vi "Rotation.vi"(1 "Uncorrected Speed":dbl=-0.0, 2 "Moving Laterally":bool) -> (0 "Output Speed":dbl=-0.0)   [LabVIEW 2013]
uses:
  Robot Global Data.vi
panel:
  in  "Output Range":cluster{"output high":dbl, "output low":dbl}={"output high"=0.4, "output low"=-0.4}
  in  "Gain":dbl=0.02
  in  "Rate Limit (deg/s)":dbl=15.0
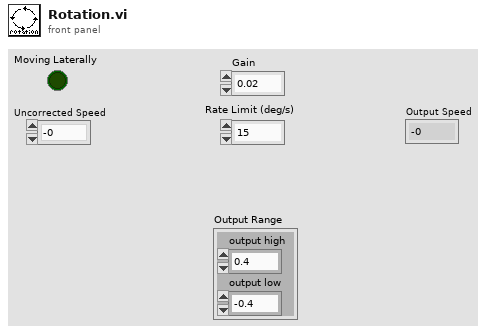
[diagram p1: front panel]
types:
  T1 = typedef "WPI_GyroDevRef.ctl" = cluster{"DevStatus":errorcluster, "Analog Module":T2, "Analog Channel":T3, "Offset":dbl, "Gain (VoltsPerDegree/Second)":dbl}
  T2 = typedef "FPGA_TypedefAnalogModule.ctl" = enum16{"Analog Module 1", "Analog Module 2"}
  T3 = typedef "FPGA_AIChannel.ctl" = enum8{"AI 1", "AI 2", "AI 3", "AI 4", "AI 5", "AI 6", "AI 7", "AI 8", "Invalid"}
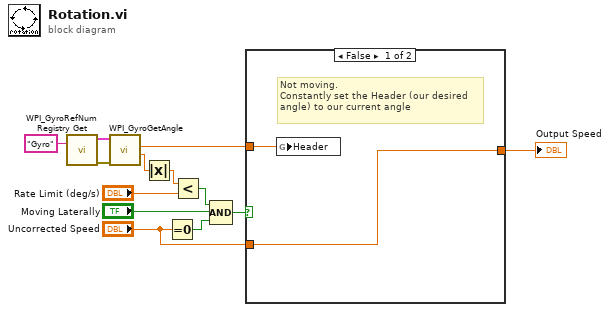
[diagram p0: block diagram]
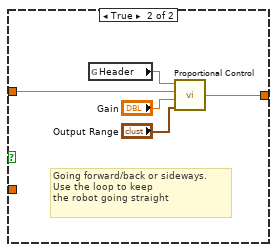
[diagram p2: hidden frame]
diagram:
  n1 = call <vilib>:"WPI_GyroRefNum Registry Get.vi"("refnum name"="Gyro") -> ("error out"=w5:errorcluster, "GyroDevRef"=w12:T1)  [unwired: 9 in]
  n2 = call <vilib>:"WPI_GyroGetAngle.vi"("error in (no error)"=w5, "GyroDevRef"=w12) -> ("Angular Rate"=w8:dbl, "Angle"=w11:dbl)  [unwired: 6 in, 2 out]
  n3 = Absolute Value(x=w8) -> (abs(x)=w4:dbl)
  n4 = Equal To 0?(x="Uncorrected Speed") -> (x = 0?=w2:bool)
  n5 = Less?(x=w4, y="Rate Limit (deg/s)") -> (x < y?=w7:bool)
  n6 = Compound Arithmetic op=AND(w7, "Moving Laterally", w2) -> (w6:bool)
  n7 = case shown="False" w6 {
    tunnel: "Uncorrected Speed" -> [w15 _]
    tunnel: [w15 w16] -> w9
    tunnel: w11 -> [w14 w20]
    frame False {
      # "Not moving.\nConstantly set the Header (our desired\nangle) to our current angle"
      n8 = global write "Robot Global Data.vi" "Header"(w14) -> ()
    }
    frame True {
      # "Going forward/back or sideways.\nUse the loop to keep \nthe robot going straight"
      n9 = global read "Robot Global Data.vi" "Header"() -> (w19:dbl)
      n10 = call "Proportional Control.vi"("Output Range"="Output Range", "Gain"="Gain", "Process Variable"=w20, "Setpoint"=w19) -> ("Output"=w16:dbl)  [unwired: 2 in]
    }
  }
  "Output Speed" <- w9
